vi "Set_Tunnel_Speed_server.vi"(4 "Tunnel Velocity m/s":dbl min=0.0 max=50.0 format="%.2f", 5 "Rig Name":string, 6 "Mode":T1, 7 "Client Name":string="G3_3 HD") -> (0 "Error String":string, 1 "Settling Time (s)":dbl format="%.2f", 2 "Max allowable Tunnel Velocity":dbl, 3 "Valid Client":bool)   [LabVIEW 2017]
uses:
  ADAM Client/Sub VIs/ADAM Controls/Tunnel_speed_mode.ctl
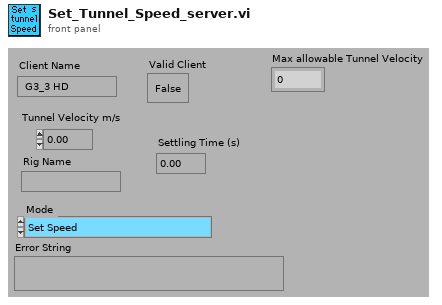
[diagram p1: front panel]
types:
  T1 = typedef "Tunnel_speed_mode.ctl" = enum16{"Set Speed", "Set Speed then wait", "Is tunnel speed allowable?"}
  T2 = typedef "Ch_description_ADAM.ctl" = cluster{"Ch Name":string, "Type":T3, "Function":T4, "Ch State":T5, "Calibration type":T6, "A":dbl, "B":dbl, "C":dbl, "D":dbl, "Comments":string, "Address":T7, "String":string, "Duty":u16}
  T3 = typedef "Module_type_ADAM.ctl" = string
  T4 = typedef "Function_ADAM.ctl" = enum16{"Analogue Input", "Digital Input", "Event counter", "Event rate", "Analogue Output", "Digital Output", "Relay Output"}
  T5 = typedef "Channel_State.ctl" = enum16{"On", "Off", "Always On", "Always Off"}
  T6 = typedef "Calib_type_ADAM.ctl" = string
  T7 = typedef "Address.ctl" = cluster{"Main":i32, "Ch.":i32, "Sub":i32, "Port Name":string}
  T8 = cluster{"Bus Bar":string, "Connected Items":string[]}
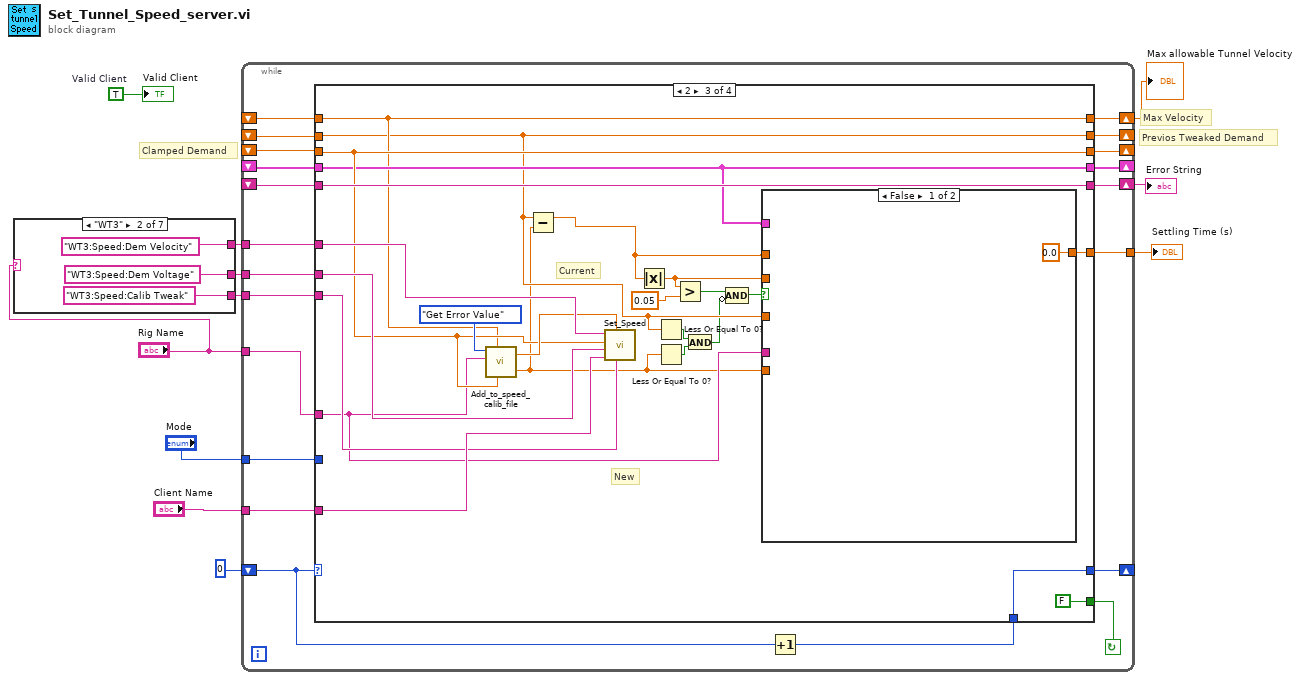
[diagram p0: block diagram]
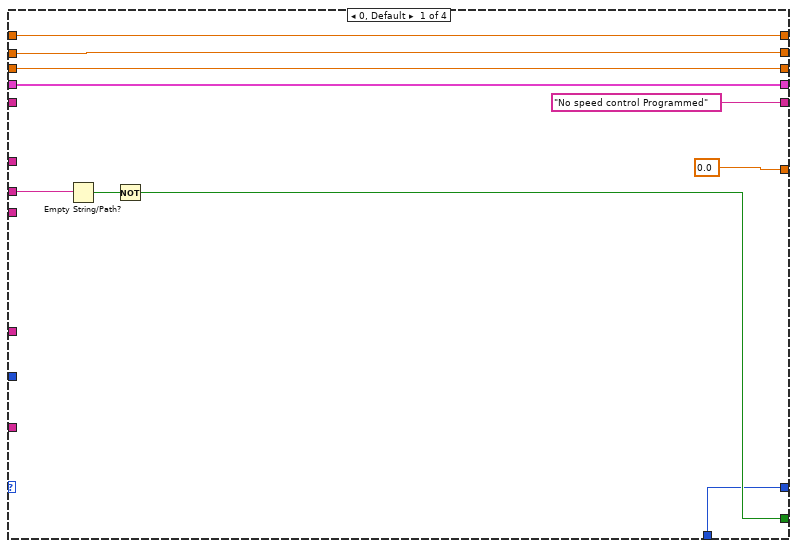
[diagram p2: hidden frame]
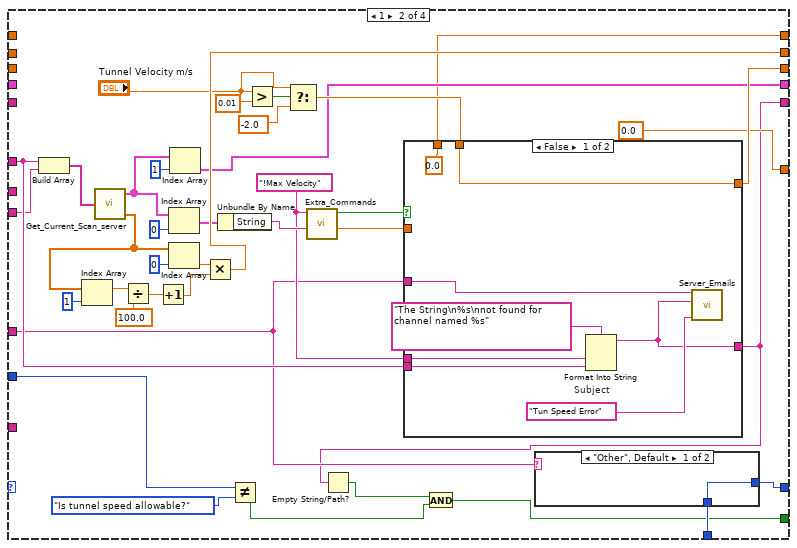
[diagram p3: hidden frame]
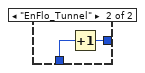
[diagram p4: hidden frame]
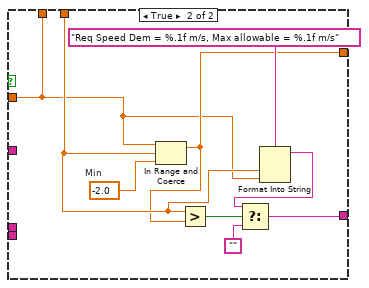
[diagram p5: hidden frame]
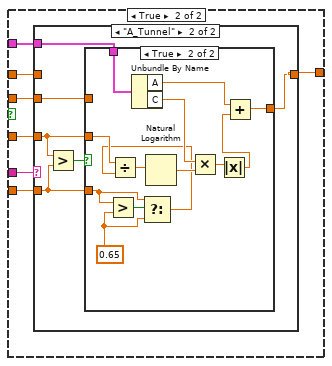
[diagram p6: hidden frame]
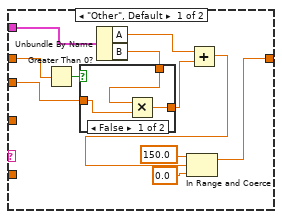
[diagram p7: hidden frame]
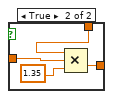
[diagram p8: hidden frame]
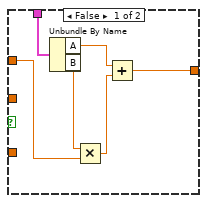
[diagram p9: hidden frame]
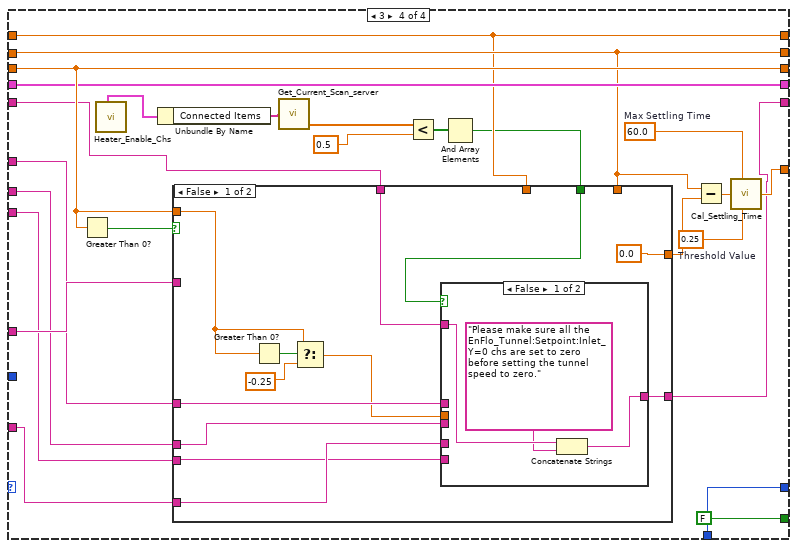
[diagram p10: hidden frame]
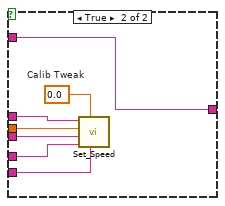
[diagram p11: hidden frame]
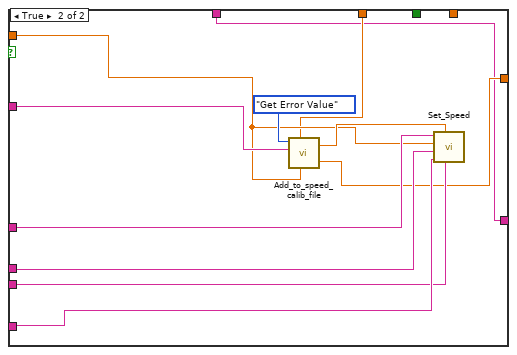
[diagram p12: hidden frame]
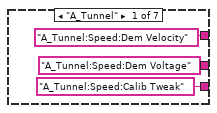
[diagram p13: hidden frame]
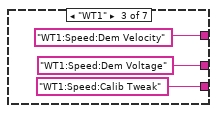
[diagram p14: hidden frame]
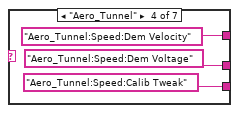
[diagram p15: hidden frame]
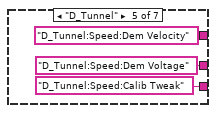
[diagram p16: hidden frame]
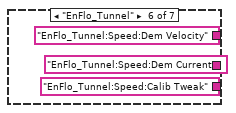
[diagram p17: hidden frame]
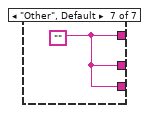
[diagram p18: hidden frame]
diagram:
  w11 = TRUE  # Valid Client
  # "Max Velocity"
  # "Previos Tweaked Demand"
  # "Clamped Demand"
  n1 = case shown="\"WT3\"" "Rig Name" {
    tunnel: ["A_Tunnel:Speed:Dem Velocity" "WT3:Speed:Dem Velocity" "WT1:Speed:Dem Velocity" "Aero_Tunnel:Speed:Dem Velocity" "D_Tunnel:Speed:Dem Velocity" "EnFlo_Tunnel:Speed:Dem Velocity" w30] -> w7
    tunnel: ["A_Tunnel:Speed:Dem Voltage" "WT3:Speed:Dem Voltage" "WT1:Speed:Dem Voltage" "Aero_Tunnel:Speed:Dem Voltage" "D_Tunnel:Speed:Dem Voltage" "EnFlo_Tunnel:Speed:Dem Current" w30] -> w4
    tunnel: ["A_Tunnel:Speed:Calib Tweak" "WT3:Speed:Calib Tweak" "WT1:Speed:Calib Tweak" "Aero_Tunnel:Speed:Calib Tweak" "D_Tunnel:Speed:Calib Tweak" "EnFlo_Tunnel:Speed:Calib Tweak" w30] -> w2
    frame "A_Tunnel" {
    }
    frame "WT3" {
    }
    frame "WT1" {
    }
    frame "Aero_Tunnel" {
    }
    frame "D_Tunnel" {
    }
    frame "EnFlo_Tunnel" {
    }
    frame "Other", Default {
      w30 = ""
    }
  }
  n2 = while {
    shift-left: _ -> [w33]
    shift-right: [w34] -> _
    tunnel: w2 -> [w35]
    shift-left: _ -> [w37]
    shift-right: [w36] -> _
    tunnel: [w38] -> w3
    tunnel: w4 -> [w40]
    shift-left: _ -> [w39]
    shift-right: [w43] -> w6
    shift-left: _ -> [w41]
    shift-right: [w44] -> _
    tunnel: w7 -> [w45]
    shift-left: 0 -> [w48]
    shift-right: [w47] -> _
    tunnel: "Client Name" -> [w50]
    tunnel: "Mode" -> [w51]
    tunnel: "Rig Name" -> [w49]
    shift-right: [w32] -> w1
    shift-left: _ -> [w31]
    stop <- w42 continue-if-true
    n3 = Increment(x=w48) -> (x+1=w46:i32)
    n4 = case shown="2" w48 {
      tunnel: w41 -> [w57 _ w134 w211]
      tunnel: w51 -> [_ w90 _ _]
      tunnel: ["No speed control Programmed" w63 w138 w200] -> w43
      tunnel: w50 -> [_ _ w143 w218]
      tunnel: w49 -> [_ w82 w130 w217]
      tunnel: [w58 w85 w141 w212] -> w47
      tunnel: w46 -> [w58 w86 w141 w212]
      tunnel: w45 -> [_ w94 w140 w215]
      tunnel: [w57 w92 w134 w211] -> w44
      tunnel: [w59 w62 FALSE FALSE] -> w42
      tunnel: w40 -> [w61 _ w139 w214]
      tunnel: w39 -> [_ _ w138 w201]
      tunnel: [0.0 ("Settling Time") 0.0 ("Settling Time") w133 w209] -> w38
      tunnel: w37 -> [w55 _ w126 w204]
      tunnel: [w55 w73 w126 w204] -> w36
      tunnel: w35 -> [_ w81 w136 w207]
      tunnel: [w53 w67 w132 w205] -> w34
      tunnel: w33 -> [w53 _ w132 w205]
      tunnel: [w52 w66 w129 w203] -> w32
      tunnel: w31 -> [w52 _ w129 w203]
      frame 0, Default {
        n5 = Empty String/Path?(string/path=w61) -> (empty?=w60:bool)
        n6 = Not(x=w60) -> (.not. x?=w59:bool)
      }
      frame 1 {
        w95 = "!Max Velocity" ("Command")
        n7 = Build Array(w94, w81) -> (w99:string[])
        n8 = call "Get_Current_Scan_server.vi"("Desired Channels"=w99) -> ("Ch Description Array"=w68:T2[], "Numerical Values"=w79:dbl[])  [unwired: 1 out]
        n9 = Index Array(array=w79, index=1 ("Index")) -> (element=w78:dbl)
        n10 = Divide(x=w78, y=100.0) -> (x/y=w76:dbl)
        n11 = Increment(x=w76) -> (x+1=w74:dbl)
        n12 = Index Array(array=w68, index=0 ("Index")) -> (element=w70:T2)
        n13 = Index Array(array=w79, index=0 ("Index")) -> (element=w75:dbl)
        n14 = Index Array(array=w68, index=1 ("Index")) -> (element=w67:T2)
        n15 = Multiply(x=w75, y=w74) -> (x*y=w73:dbl)
        n16 = Unbundle By Name(w70) -> ("String"=w97:string)
        n17 = Not Equal?(x=w90, y=Tunnel_speed_mode."Is tunnel speed allowable?" ("Mode")) -> (x != y?=w64:bool)
        n18 = Greater?(x="Tunnel Velocity m/s", y=0.01) -> (0:w89:bool)
        n19 = Select(t="Tunnel Velocity m/s", s=w89, f=-2.0 ("t")) -> (s? t:f=w87:dbl)
        n20 = call "Extra_Commands.vi"("String to Search"=w97, "Command"=w95) -> ("Numeric Value"=w93:dbl, "Command Found"=w96:bool)  [unwired: 1 in, 3 out]
        n21 = case shown="False" w96 {
          tunnel: w82 -> [w104 _]
          tunnel: w95 -> [w109 _]
          tunnel: w94 -> [w108 _]
          tunnel: w93 -> [_ w111]
          tunnel: w87 -> [w106 w113]
          tunnel: [w106 w112] -> w92
          tunnel: [w105 w115] -> w63
          tunnel: [0.0 ("Numeric Value") w111] -> w66
          frame False {
            w110 = "Tun Speed Error"  # Subject
            n22 = Format Into String(format string="The String\n%s\nnot found for channel named %s" ("Format String"), w109, w108) -> (resulting string=w105:string)  [unwired: 2 in, 1 out]
            n23 = call "Server_Emails.vi"("Client Name Contains"=w104, "Message"=w105, "Subject"=w110) -> ()  [unwired: 2 in, 3 out]
          }
          frame True {
            w119 = -2.0  # Min
            n24 = In Range and Coerce(upper limit=w111, x=w113, lower limit=w119) -> (coerced(x)=w112:dbl)  [unwired: 1 out]
            n25 = Greater?(x=w113, y=w112) -> (0:w114:bool)
            n26 = Format Into String(format string="Req Speed Dem = %.1f m/s, Max allowable = %.1f m/s", w113, w111) -> (resulting string=w117:string)  [unwired: 2 in, 1 out]
            n27 = Select(t=w117, s=w114, f="") -> (s? t:f=w115:string)
          }
        }
        n28 = Empty String/Path?(string/path=w63) -> (empty?=w65:bool)
        n29 = And(x=w65, y=w64) -> (x .and. y?=w62:bool)
        n30 = case shown="\"Other\", Default" w82 {
          tunnel: w86 -> [w100 w102]
          tunnel: [w100 w101] -> w85
          frame "Other", Default {
          }
          frame "EnFlo_Tunnel" {
            n31 = Increment(x=w102) -> (x+1=w101:i32)
          }
        }
      }
      frame 2 {
        # "Current"
        # "New"
        n32 = call "Add_to_speed_calib_file.vi"("Desired Velocity"=w134, "Max Velocity"=w129, "Rig Name"=w130, "Mode"=enum16{"Add Row", "Get Error Value"}."Get Error Value") -> ("Tweaked Demand"=w125:dbl, "Calib Tweak %"=w135:dbl)  [unwired: 2 in]
        n33 = Subtract(x=w126, y=w125) -> (x-y=w131:dbl)
        n34 = call "Set_Speed.vi"("Channel Name (Calib Tweak)"=w136, "Calib Tweak"=w135, "Client Name"=w143, "Channel Name (Volts/Amps)"=w139, "Demanded Velocity"=w134, "Channel Name (Velocity)"=w140) -> ()  [unwired: 1 in, 4 out]
        n35 = Absolute Value(x=w131) -> (abs(x)=w128:dbl)
        n36 = Less Or Equal To 0?(x=w126) -> (x <= 0?=w121:bool)
        n37 = Less Or Equal To 0?(x=w125) -> (x <= 0?=w122:bool)
        n38 = Greater?(x=w128, y=0.05) -> (0:w124:bool)
        n39 = And(x=w121, y=w122) -> (x .and. y?=w120:bool)
        n40 = Compound Arithmetic op=AND(w124, invert w120) -> (w123:bool)
        n41 = case shown="False" w123 {
          tunnel: [0.0 ("Max") w151] -> w133
          tunnel: w132 -> [_ w150]
          tunnel: w131 -> [_ w149]
          tunnel: w126 -> [_ w148]
          tunnel: w125 -> [_ w147]
          tunnel: w130 -> [_ w146]
          tunnel: w128 -> [_ w145]
          frame False {
          }
          frame True {
            n42 = case shown="\"A_Tunnel\"" w146 {
              tunnel: w150 -> [w162 w174]
              tunnel: w149 -> [w157 _]
              tunnel: w145 -> [w153 w175]
              tunnel: [w152 w173] -> w151
              tunnel: w148 -> [_ w171]
              tunnel: w147 -> [_ w172]
              frame "Other", Default {
                n43 = Greater Than 0?(x=w157) -> (x > 0?=w156:bool)
                n44 = Unbundle By Name(w162) -> ("A"=w161:dbl, "B"=w155:dbl)
                n45 = case shown="False" w156 {
                  tunnel: [w165 w166] -> w154
                  tunnel: w155 -> [w164 w169]
                  tunnel: w153 -> [w163 w168]
                  frame False {
                    n46 = Multiply(x=w164, y=w163) -> (x*y=w165:dbl)
                  }
                  frame True {
                    n47 = Compound Arithmetic op=MULTIPLY(w169, w168, 1.35 ("Min")) -> (w166:dbl)
                  }
                }
                n48 = Add(x=w161, y=w154) -> (x+y=w158:dbl)
                n49 = In Range and Coerce(upper limit=150.0 ("Max"), x=w158, lower limit=0.0 ("Min")) -> (coerced(x)=w152:dbl)  [unwired: 1 out]
              }
              frame "A_Tunnel" {
                n50 = Greater?(x=w171, y=w172) -> (0:w170:bool)
                n51 = case shown="True" w170 {
                  tunnel: w175 -> [w177 _]
                  tunnel: w174 -> [w181 w194]
                  tunnel: [w176 w186] -> w173
                  tunnel: w171 -> [_ w192]
                  tunnel: w172 -> [_ w184]
                  frame False {
                    n52 = Unbundle By Name(w181) -> ("A"=w180:dbl, "B"=w178:dbl)
                    n53 = Multiply(x=w178, y=w177) -> (x*y=w179:dbl)
                    n54 = Add(x=w180, y=w179) -> (x+y=w176:dbl)
                  }
                  frame True {
                    w183 = 0.65 ("y")
                    n55 = Greater?(x=w184, y=w183) -> (0:w185:bool)
                    n56 = Unbundle By Name(w194) -> ("A"=w187:dbl, "C"=w190:dbl)
                    n57 = Select(t=w184, s=w185, f=w183) -> (s? t:f=w182:dbl)
                    n58 = Divide(x=w192, y=w182) -> (x/y=w193:dbl)
                    n59 = Natural Logarithm(1:w193) -> (0:w191:dbl)
                    n60 = Multiply(x=w190, y=w191) -> (x*y=w189:dbl)
                    n61 = Absolute Value(x=w189) -> (abs(x)=w188:dbl)
                    n62 = Add(x=w187, y=w188) -> (x+y=w186:dbl)
                  }
                }
              }
            }
          }
        }
      }
      frame 3 {
        w210 = 0.25  # Threshold Value
        w202 = 60.0  # Max Settling Time
        n63 = Greater Than 0?(x=w211) -> (x > 0?=w219:bool)
        n64 = call "Heater_Enable_Chs.vi"() -> ("Inlet Heaters"=w199:T8)  [unwired: 4 in, 5 out]
        n65 = Unbundle By Name(w199) -> ("Connected Items"=w198:string[])
        n66 = call "Get_Current_Scan_server.vi"("Desired Channels"=w198) -> ("Numerical Values"=w197:dbl[])  [unwired: 2 out]
        n67 = Less?(x=w197, y=0.5) -> (x < y?=w196:bool[])
        n68 = And Array Elements(Boolean array=w196) -> (logical AND=w195:bool)
        n69 = case shown="False" w219 {
          tunnel: w211 -> [w229 w244]
          tunnel: w215 -> [w228 w252]
          tunnel: w214 -> [w226 w251]
          tunnel: w218 -> [w225 w250]
          tunnel: w217 -> [_ w249]
          tunnel: w195 -> [w224 _]
          tunnel: [0.0 w245] -> w206
          tunnel: w207 -> [w222 w247]
          tunnel: w204 -> [_ _]
          tunnel: w203 -> [_ w243]
          tunnel: w201 -> [w221 w242]
          tunnel: [w220 w242] -> w200
          frame False {
            n70 = Greater Than 0?(x=w229) -> (x > 0?=w231:bool)
            n71 = Select(t=w229, s=w231, f=-0.25 ("t")) -> (s? t:f=w227:dbl)
            n72 = case shown="False" w224 {
              tunnel: w228 -> [_ w241]
              tunnel: w227 -> [_ w240]
              tunnel: w226 -> [_ w239]
              tunnel: w225 -> [_ w238]
              tunnel: w222 -> [_ w237]
              tunnel: w221 -> [w234 w235]
              tunnel: [w232 w235] -> w220
              frame False {
                n73 = Concatenate Strings(w234, "Please make sure all the EnFlo_Tunnel:Setpoint:Inlet_Y=0 chs are set to zero before setting the tunnel speed to zero.") -> (w232:string)
              }
              frame True {
                w236 = 0.0  # Calib Tweak
                n74 = call "Set_Speed.vi"("Channel Name (Calib Tweak)"=w237, "Calib Tweak"=w236, "Client Name"=w238, "Channel Name (Volts/Amps)"=w239, "Demanded Velocity"=w240, "Channel Name (Velocity)"=w241) -> ()  [unwired: 1 in, 4 out]
              }
            }
          }
          frame True {
            n75 = call "Add_to_speed_calib_file.vi"("Desired Velocity"=w244, "Max Velocity"=w243, "Rig Name"=w249, "Mode"=enum16{"Add Row", "Get Error Value"}."Get Error Value") -> ("Tweaked Demand"=w245:dbl, "Calib Tweak %"=w246:dbl)  [unwired: 2 in]
            n76 = call "Set_Speed.vi"("Channel Name (Calib Tweak)"=w247, "Calib Tweak"=w246, "Client Name"=w250, "Channel Name (Volts/Amps)"=w251, "Demanded Velocity"=w244, "Channel Name (Velocity)"=w252) -> ()  [unwired: 1 in, 4 out]
          }
        }
        n77 = Subtract(x=w204, y=w206) -> (x-y=w208:dbl)
        n78 = call "Cal_Settling_Time.vi"("Max Settling Time"=w202, "Speed Tweak (m/s)"=w208, "Threshold Value"=w210) -> ("Required Settling Time"=w209:dbl)  [unwired: 2 out]
      }
    }
  }
  "Error String" <- w6
  "Settling Time (s)" <- w3
  "Max allowable Tunnel Velocity" <- w1
  "Valid Client" <- w11
